vi "Remap.vi"(0 "x":dbl, 5 "In Min":dbl, 7 "In Max":dbl, 9 "Out Min":dbl, 11 "Out Max":dbl) -> (8 "y":dbl)   [LabVIEW 2021]
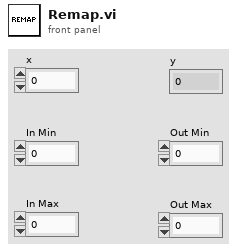
[diagram p1: front panel]
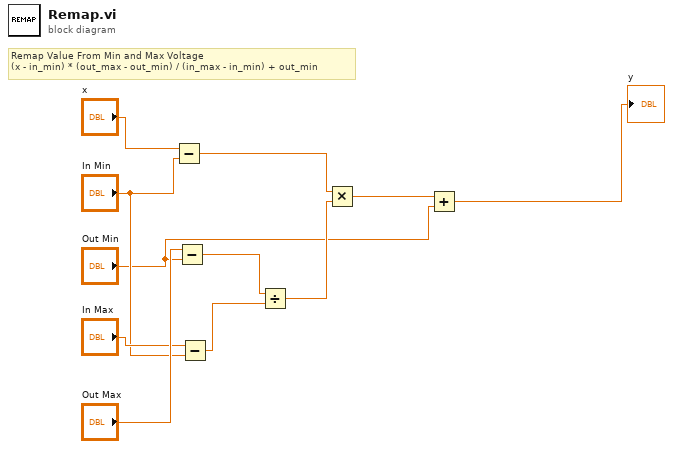
[diagram p0: block diagram]
diagram:
  # "Remap Value From Min and Max Voltage\n(x - in_min) * (out_max - out_min) / (in_max - in_min) + out_min"
  n1 = Subtract(x="x", y="In Min") -> (x-y=w5:dbl)
  n2 = Subtract(x="Out Max", y="Out Min") -> (x-y=w7:dbl)
  n3 = Subtract(x="In Max", y="In Min") -> (x-y=w6:dbl)
  n4 = Divide(x=w7, y=w6) -> (x/y=w4:dbl)
  n5 = Multiply(x=w5, y=w4) -> (x*y=w3:dbl)
  n6 = Add(x=w3, y="Out Min") -> (x+y=→"y":dbl)
